vi "Control value mapping.vi"(1 "Control In%":dbl, 2 "Demand Out%":dbl[](array[numeric]), 3 "Demand In%":dbl[](array[numeric])) -> (0 "Control Out%":dbl)   [LabVIEW 2022 SP3]
uses:
  <vilib>/Analysis/NI_AALPro.lvlib
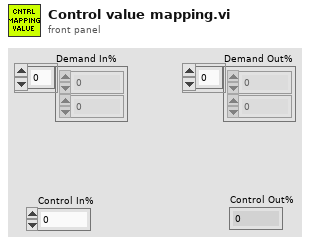
[diagram p1: front panel]
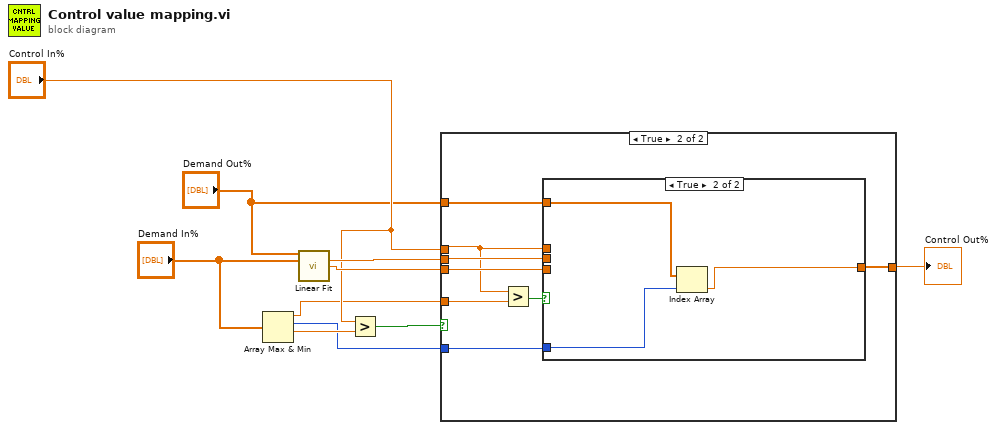
[diagram p0: block diagram]
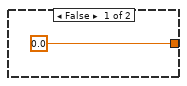
[diagram p2: hidden frame]
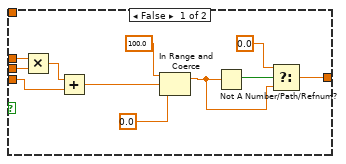
[diagram p3: hidden frame]
diagram:
  n1 = Array Max & Min(array="Demand In%") -> (max value=w3:dbl, max index (indices)=w2:i32, min value=w5:dbl)  [unwired: 1 out]
  n2 = call <vilib>:"Linear Fit.vi"("Y"="Demand Out%", "X"="Demand In%") -> ("slope"=w10:dbl, "intercept"=w9:dbl)  [unwired: 9 in, 3 out]
  n3 = Greater?(x="Control In%", y=w5) -> (0:w4:bool)
  n4 = case shown="True" w4 {
    tunnel: w10 -> [_ w19]
    tunnel: w9 -> [_ w18]
    tunnel: [0.0 ("upper limit") w17] -> w8
    tunnel: "Control In%" -> [_ w16]
    tunnel: w3 -> [_ w15]
    tunnel: w2 -> [_ w13]
    tunnel: "Demand Out%" -> [_ w12]
    frame False {
    }
    frame True {
      n5 = Greater?(x=w16, y=w15) -> (0:w14:bool)
      n6 = case shown="True" w14 {
        tunnel: w19 -> [w30 _]
        tunnel: w18 -> [w28 _]
        tunnel: [w21 w31] -> w17
        tunnel: w16 -> [w20 _]
        tunnel: w13 -> [_ w33]
        tunnel: w12 -> [_ w32]
        frame False {
          n7 = Multiply(x=w20, y=w30) -> (x*y=w29:dbl)
          n8 = Add(x=w29, y=w28) -> (x+y=w27:dbl)
          n9 = In Range and Coerce(upper limit=100.0, x=w27, lower limit=0.0) -> (coerced(x)=w23:dbl)  [unwired: 1 out]
          n10 = Not A Number/Path/Refnum?(number/path/refnum=w23) -> (NaN/Path/Refnum?=w24:bool)
          n11 = Select(t=0.0, s=w24, f=w23) -> (s? t:f=w21:dbl)
        }
        frame True {
          n12 = Index Array(array=w32, index=w33) -> (element=w31:dbl)
        }
      }
    }
  }
  "Control Out%" <- w8
